vi "Create Gradient Rect.vi"(6 "Color":u32(colorbox), 8 "error in (no error)":errorcluster, 9 "Size":cluster{"Width":i32, "Height":i32}={"Width"=10, "Height"=10}, 10 "Position":cluster{"Left":i32, "Top":i32}, 11 "Gradient Rectangle in":refnum<class "Gradient Rectangle.lvclass">) -> (0 "error out":errorcluster, 3 "Gradient Rectangle out":refnum<class "Gradient Rectangle.lvclass">)   [LabVIEW 2017, in "Gradient Rectangle.lvclass"]
uses:
  Gradient Rectangle.lvclass
  C:/Program Files (x86)/National Instruments/LabVIEW 2017/vi.lib/LIEF/Forms/Shape/Shape.lvclass
  C:/Program Files (x86)/National Instruments/LabVIEW 2017/vi.lib/LIEF/Forms/Layered Shape/Layered Shape.lvclass
  Gradient Rectangle.lvclass/Gradient Rectangle.ctl
  <vilib>/LIEF/Forms/Shape/Shape.lvclass/Shape.ctl
  <vilib>/LIEF/Forms/Shape/Write Color.vi
  <vilib>/LIEF/Forms/Shape/Write Movable.vi
  <vilib>/LIEF/Forms/Shape/Write Selectable.vi
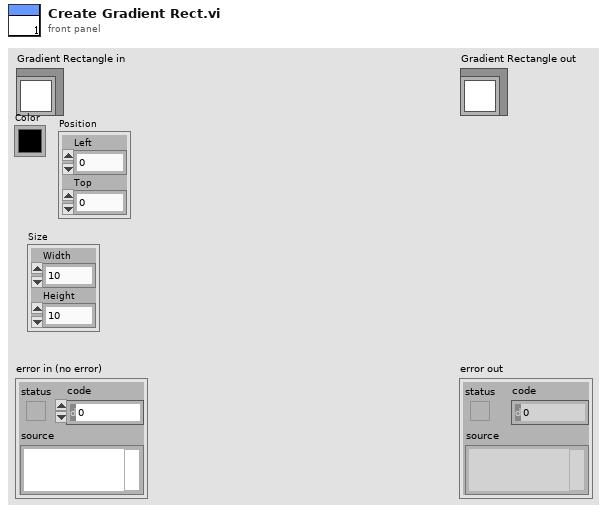
[diagram p1: front panel]
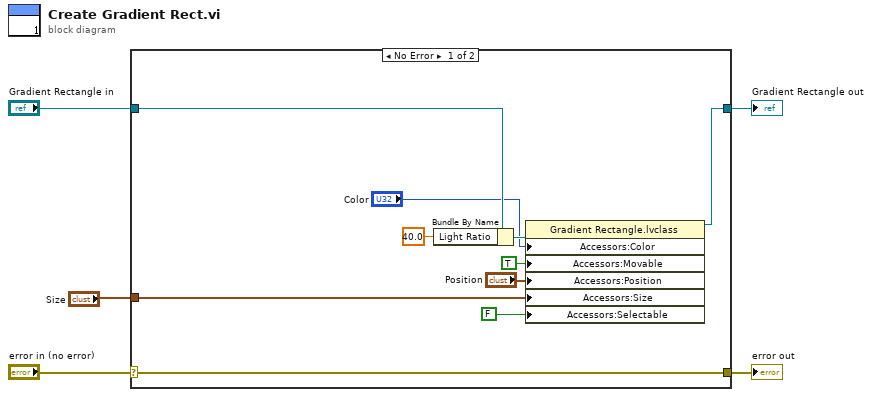
[diagram p0: block diagram]
diagram:
  n1 = case shown="No Error" "error in (no error)" {
    selector: "error in (no error)" -> [w15 w17]
    tunnel: [w15 w17] -> w4
    tunnel: [w8 w16] -> w2
    tunnel: "Gradient Rectangle in" -> [w14 w16]
    tunnel: "Size" -> [w6 _]
    frame No Error {
      n2 = Bundle By Name(cluster=w14, "Light Ratio"=40.0) -> (w12:refnum<class "Gradient Rectangle.lvclass">)
      n3 = property class="Gradient Rectangle.lvclass"(reference=w12, "Accessors:Color"="Color", "Accessors:Movable"=TRUE ("Movable"), "Accessors:Position"="Position", "Accessors:Size"=w6, "Accessors:Selectable"=FALSE ("Selectable")) -> (reference out=w8:refnum<class "Gradient Rectangle.lvclass">)  [unwired: 1 in, 1 out]
    }
    frame Error {
    }
  }
  "error out" <- w4
  "Gradient Rectangle out" <- w2
